vi "HandleStatement.vi"(7 "Statement":T1={"timestamp"=timestamp(0 s since 1904-01-01), "level"=enum."INFO", "sourceTag"="", "originVI"="", "message"=""}, 8 "error in (no error)":errorcluster, 11 "Appender in":refnum<class "Appender.lvclass">) -> (0 "error out":errorcluster, 3 "Appender out":refnum<class "Appender.lvclass">)   [LabVIEW 2026, in "Lumberjack.lvlib" / "Appender.lvclass"]
doc: "Apply the appender's own acceptance logic to one Statement: first the per-appender threshold (RankCompare against config.threshold), then the Filter (mirror accepts all above threshold; routed accepts only within the level range and matching the source-tag prefix). On acceptance, call the dynamic-dispatch Write with the Statement; on rejection, do nothing. Does not format (Write does) and does not handle queue backpressure (that is the Actor Core intake path). Static; protected (SRS-LMBR-009, 026, 027)."
uses:
  Appender.lvclass
  TypeDefs/Statement.ctl
  TypeDefs/Severity.ctl
  Appender.lvclass/Appender.ctl
  Lumberjack.lvlib
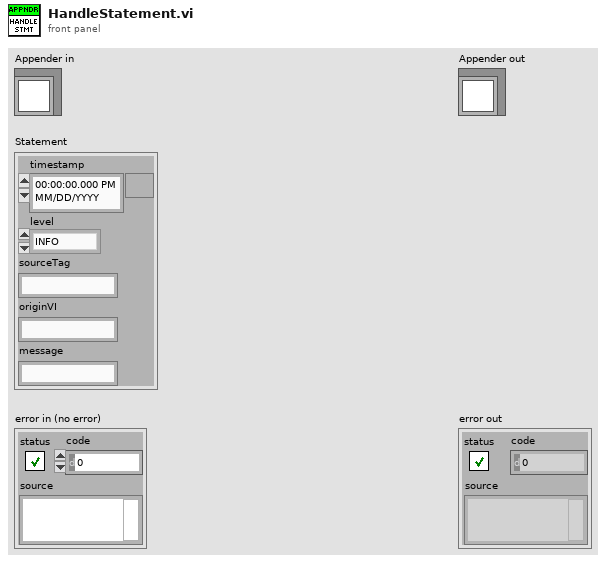
[diagram p1: front panel]
types:
  T1 = typedef "Lumberjack.lvlib/Statement.ctl" = cluster{"timestamp":timestamp, "level":T2, "sourceTag":string, "originVI":string, "message":string}
  T2 = typedef "Lumberjack.lvlib/Severity.ctl" = enum16{"OFF", "FATAL", "ERROR", "WARN", "INFO", "DEBUG", "TRACE", "ALL"}
  T3 = typedef "Lumberjack.lvlib/Filter.ctl" = cluster{"mode":T4, "levelMin":T2, "levelMax":T2, "tagPrefix":string}
  T4 = typedef "Lumberjack.lvlib/FilterMode.ctl" = enum16{"Mirror", "Routed"}
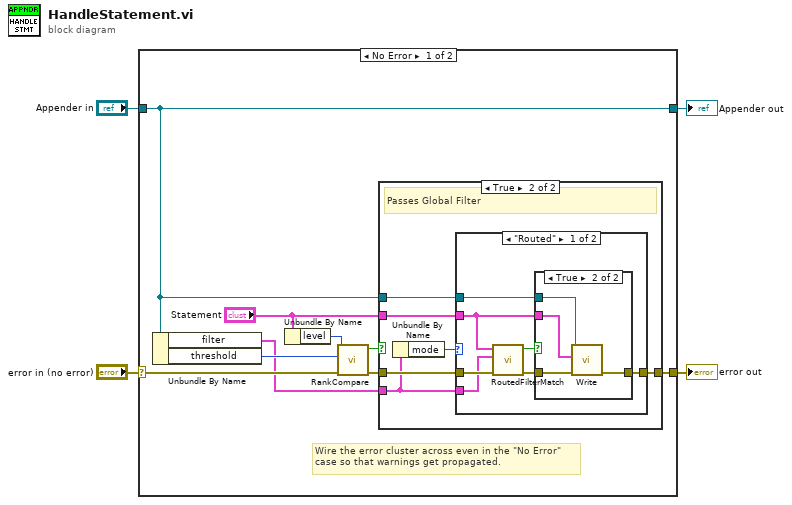
[diagram p0: block diagram]
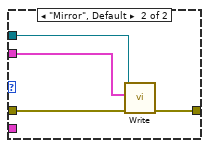
[diagram p4: hidden frame]
diagram:
  n1 = case shown="No Error" "error in (no error)" {
    selector: "error in (no error)" -> [w13 w38]
    tunnel: [w9 w38] -> w3
    tunnel: [w6 w37] -> w1
    tunnel: "Appender in" -> [w6 w37]
    frame No Error {
      # "Wire the error cluster across even in the \"No Error\"\ncase so that warnings get propagated."
      n2 = Unbundle By Name(w6) -> ("filter"=w8:T3, "threshold"=w12:T2)
      n3 = Unbundle By Name("Statement") -> ("level"=w5:T2)
      n4 = call "RankCompare.vi"("error in (no error)"=w13, "Threshold"=w12, "Level"=w5) -> ("error out"=w10:errorcluster, "Passes"=w7:bool)  [unwired: 7 in]
      n5 = case shown="True" w7 {
        tunnel: "Statement" -> [_ w20]
        tunnel: w10 -> [w14 w19]
        tunnel: [w14 w18] -> w9
        tunnel: w8 -> [_ w16]
        tunnel: w6 -> [_ w17]
        frame False {
          # "Fails Global Filter"
        }
        frame True {
          # "Passes Global Filter"
          n6 = Unbundle By Name(w16) -> ("mode"=w15:T4)
          n7 = case shown="\"Routed\"" w15 {
            tunnel: w20 -> [w21 w34]
            tunnel: w19 -> [w25 w33]
            tunnel: [w27 w36] -> w18
            tunnel: w17 -> [w26 w35]
            tunnel: w16 -> [w23 _]
            frame "Routed" {
              n8 = call "RoutedFilterMatch.vi"("error in (no error)"=w25, "Filter"=w23, "Statement"=w21) -> ("error out"=w24:errorcluster, "Accepted"=w22:bool)  [unwired: 7 in]
              n9 = case shown="True" w22 {
                tunnel: w24 -> [w28 w32]
                tunnel: [w28 w31] -> w27
                tunnel: w26 -> [_ w30]
                tunnel: w21 -> [_ w29]
                frame False {
                }
                frame True {
                  n10 = call-dynamic "Write.vi"("error in (no error)"=w32, "Statement"=w29, "Appender in"=w30) -> ("error out"=w31:errorcluster)  [unwired: 7 in, 1 out]
                }
              }
            }
            frame "Mirror", Default {
              n11 = call-dynamic "Write.vi"("error in (no error)"=w33, "Statement"=w34, "Appender in"=w35) -> ("error out"=w36:errorcluster)  [unwired: 7 in, 1 out]
            }
          }
        }
      }
    }
    frame Error {
    }
  }
  "error out" <- w3
  "Appender out" <- w1
